vi "Create Pulse Output.vi"(8 "error in (no error)":errorcluster, 10 "Params":variant, 11 "Counter Output in":refnum<class "Counter Output.lvclass">) -> (0 "error out":errorcluster, 3 "Counter Output out":refnum<class "Counter Output.lvclass">)   [LabVIEW 2020, in "Instrument.lvlib" / "Counter Output.lvclass"]
uses:
  Counter Output.lvclass
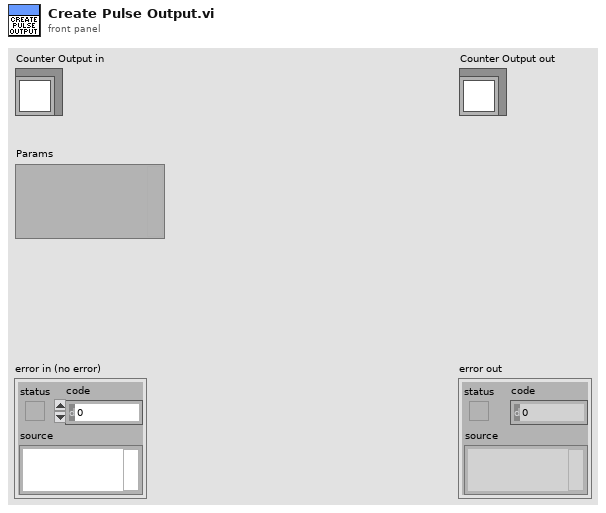
[diagram p1: front panel]
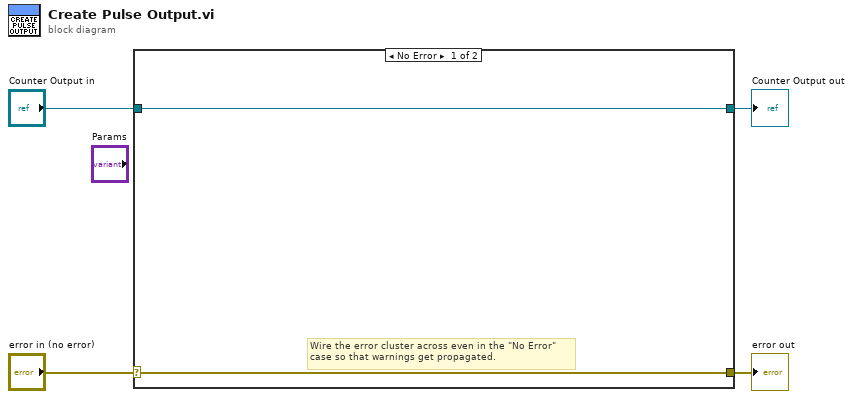
[diagram p0: block diagram]
diagram:
  n1 = case shown="No Error" "error in (no error)" {
    selector: "error in (no error)" -> [w5 w8]
    tunnel: [w5 w8] -> w3
    tunnel: [w6 w7] -> w1
    tunnel: "Counter Output in" -> [w6 w7]
    frame No Error {
      # "Wire the error cluster across even in the \"No Error\"\ncase so that warnings get propagated."
    }
    frame Error {
    }
  }
  "error out" <- w3
  "Counter Output out" <- w1
